vi "throw error if cancelled.vi"(8 "error in":errorcluster, 10 "code":i32=42, 11 "task token in":refnum<class "null task token.lvclass">) -> (0 "error out":errorcluster, 3 "task token out":refnum<class "null task token.lvclass">)   [LabVIEW 2013, in "null task token.lvclass"]
uses:
  null task token.lvclass
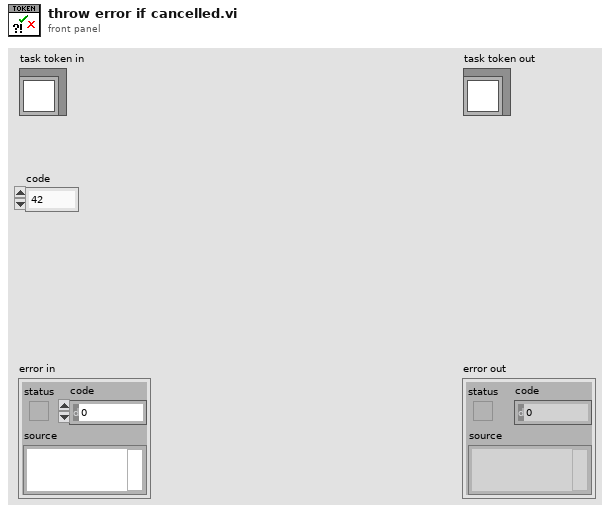
[diagram p1: front panel]
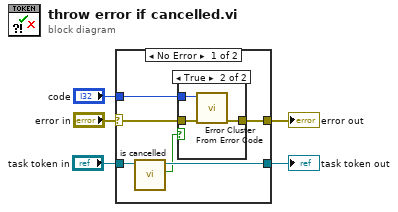
[diagram p0: block diagram]
diagram:
  n1 = case shown="No Error" "error in" {
    selector: "error in" -> [w10 w17]
    tunnel: [w8 w17] -> w4
    tunnel: [w9 w16] -> w2
    tunnel: "task token in" -> [w11 w16]
    tunnel: "code" -> [w6 _]
    frame No Error {
      n2 = call-dynamic "is cancelled.vi"("null task token in"=w11) -> ("cancelled?"=w7:bool, "null task token out"=w9:refnum<class "null task token.lvclass">)  [unwired: 9 in]
      n3 = case shown="True" w7 {
        tunnel: w10 -> [w12 w15]
        tunnel: [w12 w14] -> w8
        tunnel: w6 -> [_ w13]
        frame False {
        }
        frame True {
          n4 = call <vilib>:"Error Cluster From Error Code.vi"("error in (no error)"=w15, "error code (0)"=w13) -> ("error out"=w14:errorcluster)  [unwired: 7 in]
        }
      }
    }
    frame Error {
    }
  }
  "error out" <- w4
  "task token out" <- w2
